vi "Test Query Audio Backends.vi"(8 "error in (no error)":errorcluster) -> (0 "error out":errorcluster, 3 "Pass?":bool)   [LabVIEW 2020]
uses:
  G-Audio/Controls/Backends.ctl
  G-Audio/G-Audio.lvlib
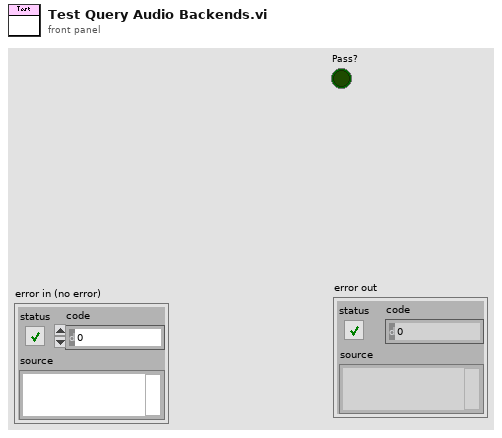
[diagram p1: front panel]
types:
  T1 = typedef "G-Audio.lvlib/Backends.ctl" = enum16{"WASAPI", "DirectSound", "WinMM", "Core Audio", "sndio", "audio(4)", "OSS", "PulseAudio", "ALSA", "JACK", "AAudio", "OpenSL|ES", "Web Audio", "Custom", "Null", "Default"}
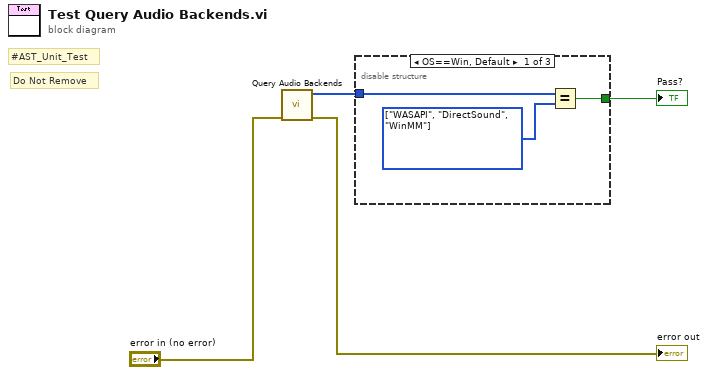
[diagram p0: block diagram]
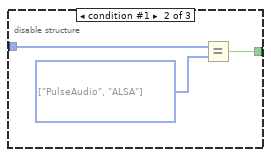
[diagram p2: hidden frame]
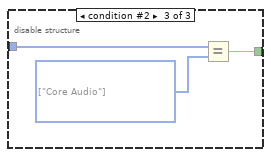
[diagram p3: hidden frame]
diagram:
  # "Do Not Remove"
  # "#AST_Unit_Test"
  n1 = call "Query Audio Backends.vi"("error in (no error)"="error in (no error)") -> ("error out"=→"error out":errorcluster, "Backends"=w3:T1[])  [unwired: 9 in]
  n2 = disable-structure shown="OS==Win, Default" {
    disable-tunnel: w3 -> [w7 w10 w13]
    disable-tunnel: [w5 w8 w11] -> w1
    frame condition #0 (active) {
      w6 = T1[] [enum."WASAPI", enum."DirectSound", enum."WinMM"] items=["WASAPI", "DirectSound", "WinMM", "Core Audio", "sndio", "audio(4)", "OSS", "PulseAudio", "ALSA", "JACK", "AAudio", "OpenSL|ES", "Web Audio", "Custom", "Null", "Default"] ("y")
      n3 = Equal?(x=w7, y=w6) -> (x = y?=w5:bool)
    }
    frame condition #1 {
      w9 = T1[] [enum."PulseAudio", enum."ALSA"] items=["WASAPI", "DirectSound", "WinMM", "Core Audio", "sndio", "audio(4)", "OSS", "PulseAudio", "ALSA", "JACK", "AAudio", "OpenSL|ES", "Web Audio", "Custom", "Null", "Default"] ("y")
      n4 = Equal?(x=w10, y=w9) -> (x = y?=w8:bool)
    }
    frame condition #2 {
      w12 = T1[] [enum."Core Audio"] items=["WASAPI", "DirectSound", "WinMM", "Core Audio", "sndio", "audio(4)", "OSS", "PulseAudio", "ALSA", "JACK", "AAudio", "OpenSL|ES", "Web Audio", "Custom", "Null", "Default"] ("y")
      n5 = Equal?(x=w13, y=w12) -> (x = y?=w11:bool)
    }
  }
  "Pass?" <- w1
